vi "HW_set_IO_ports.vi"() -> ()   [LabVIEW 2016]
panel:
  out "Sync parameters cluster output":cluster{"SYNC configuration":u32}
  in  "Reset IO":bool
  in  "IO 4 zone":bool
  in  "IO 4 start/stop":bool
  in  "IO 3 zone":bool
  in  "IO 3 start/stop":bool
  in  "IO 2 sync":bool
  in  "IO 2 zone":bool=TRUE
  in  "IO 2 start/stop":bool
  in  "IO 1 sync":bool
  in  "IO 1 zone":bool=TRUE
  in  "IO 1 start/stop":bool
  in  "IO 4":u8(slide)=1 scale=0.0..1.0
  in  "IO 3":u8(slide)=1 scale=0.0..1.0
  in  "IO 2":u8(slide) scale=0.0..1.0
  in  "Exit":bool
  in  "Save Settings":bool
  in  "IO 1":u8(slide) scale=0.0..1.0
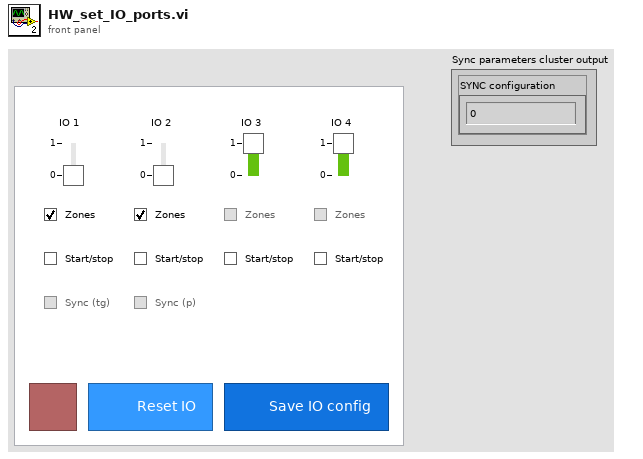
[diagram p1: front panel]
types:
  T1 = enum8{"Enabled", "Disabled", "Disabled and Grayed Out"}
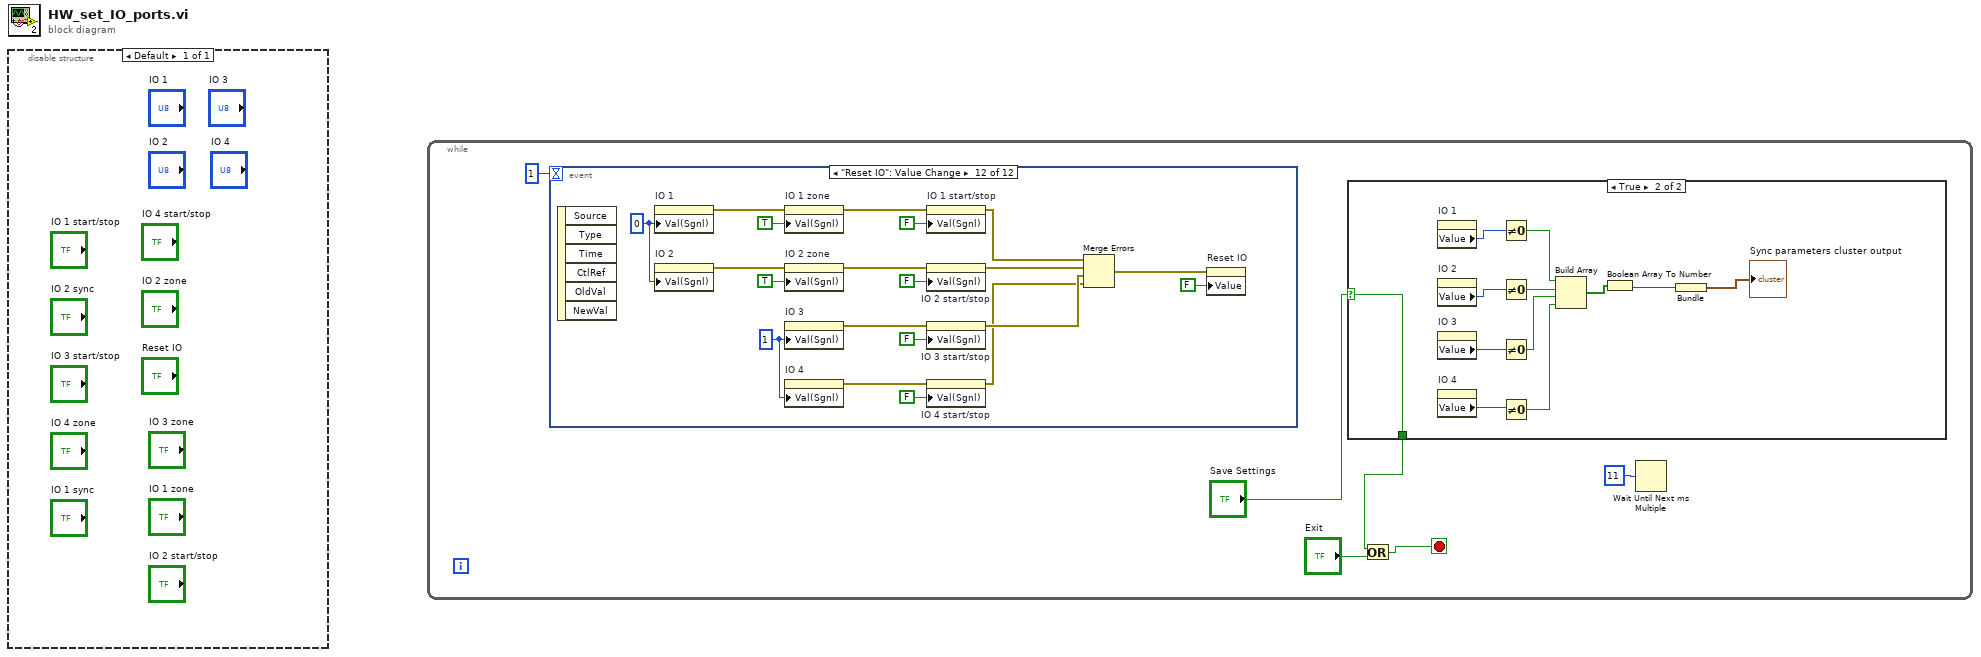
[diagram p0: block diagram]
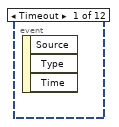
[diagram p3: hidden frame]
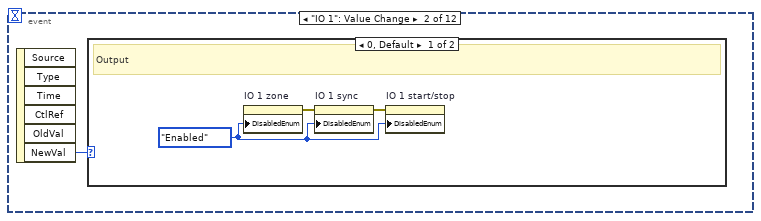
[diagram p4: hidden frame]
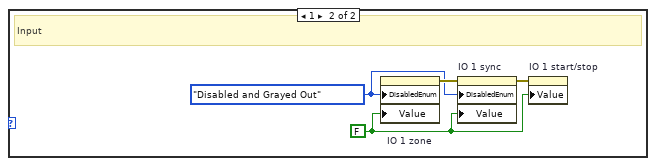
[diagram p5: hidden frame]
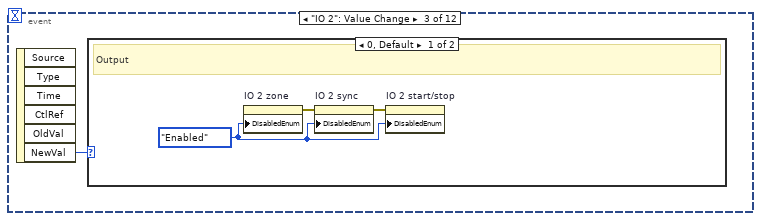
[diagram p6: hidden frame]
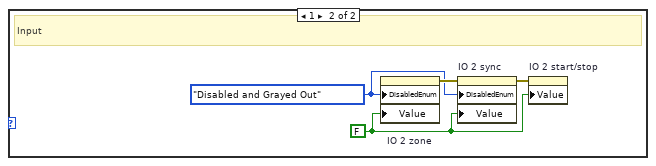
[diagram p7: hidden frame]
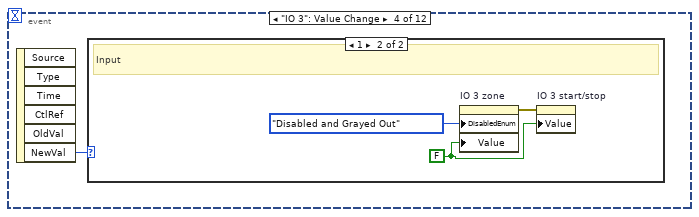
[diagram p8: hidden frame]
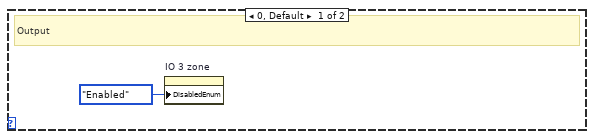
[diagram p9: hidden frame]
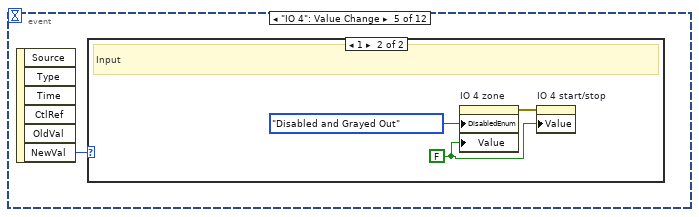
[diagram p10: hidden frame]
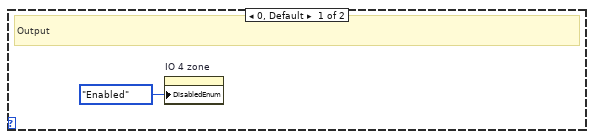
[diagram p11: hidden frame]
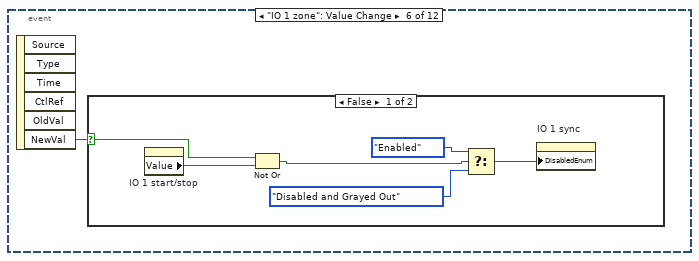
[diagram p12: hidden frame]
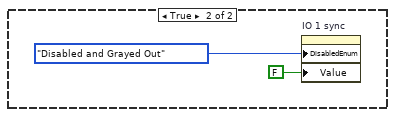
[diagram p13: hidden frame]
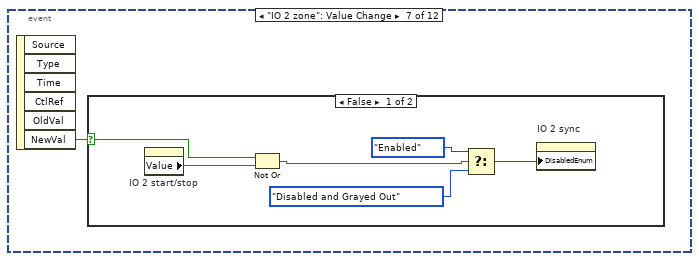
[diagram p14: hidden frame]
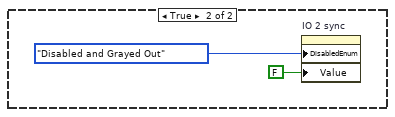
[diagram p15: hidden frame]
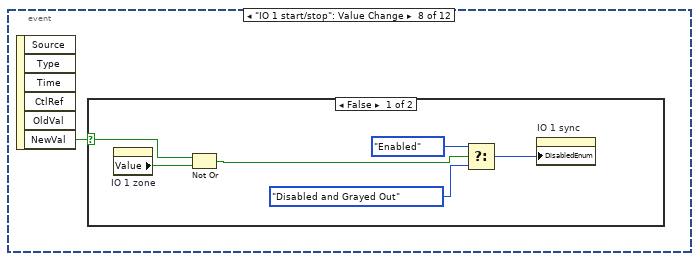
[diagram p16: hidden frame]
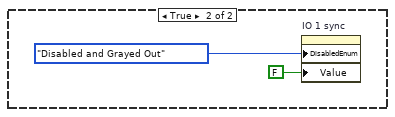
[diagram p17: hidden frame]
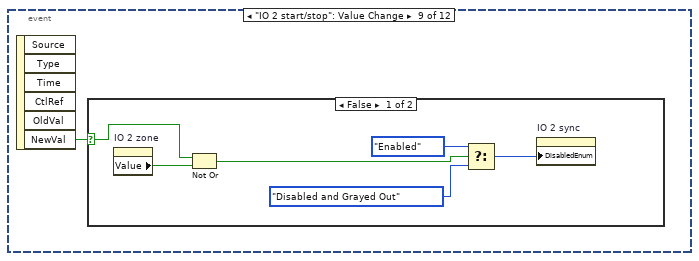
[diagram p18: hidden frame]
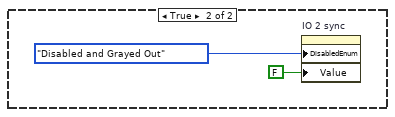
[diagram p19: hidden frame]
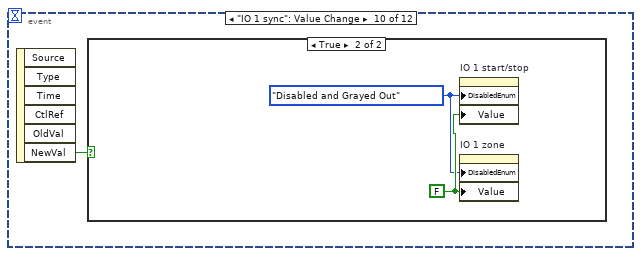
[diagram p20: hidden frame]
diagram:
  n1 = disable-structure shown="Default" {
    frame Enabled {
    }
  }
  n2 = while {
    stop <- w3 stop-if-true
    n3 = event shown="[11] \"Reset IO\": Value Change" {
      selector: _ -> [_ _ _ _ _ _ _ _ _ _ _ _]
      dyn-events: _ -> [_ _ _ _ _ _ _ _ _ _ _ _]
      timeout: 1 -> [_ _ _ _ _ _ _ _ _ _ _ _]
      event Timeout {
        n4 = event-data() -> ()  [unwired: 1 in, 3 out]
      }
      event "IO 1": Value Change {
        n5 = event-data() -> ("NewVal"=w20:u8)  [unwired: 1 in, 5 out]
        n6 = case shown="0, Default" w20 {
          frame 0, Default {
            w21 = T1."Enabled" ("Disabled")
            # "Output"
            n7 = property on="IO 1 zone" class="Bool (strict)"("DisabledEnum"=w21) -> (error out=w23:errorcluster)  [unwired: 2 in, 1 out]
            n8 = property on="IO 1 sync" class="Bool (strict)"(error in=w23, "DisabledEnum"=w21) -> (error out=w22:errorcluster)  [unwired: 1 in, 1 out]
            n9 = property on="IO 1 start/stop" class="Bool (strict)"(error in=w22, "DisabledEnum"=w21) -> ()  [unwired: 1 in, 2 out]
          }
          frame 1 {
            w24 = FALSE ("IO 1 std.")
            w26 = T1."Disabled and Grayed Out" ("Disabled")
            # "Input"
            n10 = property on="IO 1 zone" class="Bool (strict)"("DisabledEnum"=w26, "Value"=w24) -> (error out=w27:errorcluster)  [unwired: 2 in, 1 out]
            n11 = property on="IO 1 sync" class="Bool (strict)"(error in=w27, "DisabledEnum"=w26, "Value"=w24) -> (error out=w25:errorcluster)  [unwired: 1 in, 1 out]
            n12 = property on="IO 1 start/stop" class="Bool (strict)"(error in=w25, "Value"=w24) -> ()  [unwired: 1 in, 2 out]
          }
        }
      }
      event "IO 2": Value Change {
        n13 = event-data() -> ("NewVal"=w28:u8)  [unwired: 1 in, 5 out]
        n14 = case shown="0, Default" w28 {
          frame 0, Default {
            w29 = T1."Enabled" ("Disabled")
            # "Output"
            n15 = property on="IO 2 zone" class="Bool (strict)"("DisabledEnum"=w29) -> (error out=w31:errorcluster)  [unwired: 2 in, 1 out]
            n16 = property on="IO 2 sync" class="Bool (strict)"(error in=w31, "DisabledEnum"=w29) -> (error out=w30:errorcluster)  [unwired: 1 in, 1 out]
            n17 = property on="IO 2 start/stop" class="Bool (strict)"(error in=w30, "DisabledEnum"=w29) -> ()  [unwired: 1 in, 2 out]
          }
          frame 1 {
            w32 = FALSE ("IO 1 std.")
            w34 = T1."Disabled and Grayed Out" ("Disabled")
            # "Input"
            n18 = property on="IO 2 zone" class="Bool (strict)"("DisabledEnum"=w34, "Value"=w32) -> (error out=w35:errorcluster)  [unwired: 2 in, 1 out]
            n19 = property on="IO 2 sync" class="Bool (strict)"(error in=w35, "DisabledEnum"=w34, "Value"=w32) -> (error out=w33:errorcluster)  [unwired: 1 in, 1 out]
            n20 = property on="IO 2 start/stop" class="Bool (strict)"(error in=w33, "Value"=w32) -> ()  [unwired: 1 in, 2 out]
          }
        }
      }
      event "IO 3": Value Change {
        n21 = event-data() -> ("NewVal"=w36:u8)  [unwired: 1 in, 5 out]
        n22 = case shown="1" w36 {
          frame 0, Default {
            # "Output"
            n23 = property on="IO 3 zone" class="Bool (strict)"("DisabledEnum"=T1."Enabled" ("Disabled")) -> ()  [unwired: 2 in, 2 out]
          }
          frame 1 {
            w38 = FALSE ("IO 1 std.")
            # "Input"
            n24 = property on="IO 3 zone" class="Bool (strict)"("DisabledEnum"=T1."Disabled and Grayed Out" ("Disabled"), "Value"=w38) -> (error out=w39:errorcluster)  [unwired: 2 in, 1 out]
            n25 = property on="IO 3 start/stop" class="Bool (strict)"(error in=w39, "Value"=w38) -> ()  [unwired: 1 in, 2 out]
          }
        }
      }
      event "IO 4": Value Change {
        n26 = event-data() -> ("NewVal"=w41:u8)  [unwired: 1 in, 5 out]
        n27 = case shown="1" w41 {
          frame 0, Default {
            # "Output"
            n28 = property on="IO 4 zone" class="Bool (strict)"("DisabledEnum"=T1."Enabled" ("Disabled")) -> ()  [unwired: 2 in, 2 out]
          }
          frame 1 {
            w43 = FALSE ("IO 1 std.")
            # "Input"
            n29 = property on="IO 4 zone" class="Bool (strict)"("DisabledEnum"=T1."Disabled and Grayed Out" ("Disabled"), "Value"=w43) -> (error out=w44:errorcluster)  [unwired: 2 in, 1 out]
            n30 = property on="IO 4 start/stop" class="Bool (strict)"(error in=w44, "Value"=w43) -> ()  [unwired: 1 in, 2 out]
          }
        }
      }
      event "IO 1 zone": Value Change {
        n31 = event-data() -> ("NewVal"=w46:bool)  [unwired: 1 in, 5 out]
        n32 = case shown="False" w46 {
          selector: w46 -> [w51 _]
          frame False {
            n33 = property on="IO 1 start/stop" class="Bool (strict)"() -> ("Value"=w52:bool)  [unwired: 2 in, 2 out]
            n34 = Not Or(1:w52, 2:w51) -> (0:w50:bool)
            n35 = Select(t=T1."Enabled" ("Disabled"), s=w50, f=T1."Disabled and Grayed Out") -> (s? t:f=w48:T1)
            n36 = property on="IO 1 sync" class="Bool (strict)"("DisabledEnum"=w48) -> ()  [unwired: 2 in, 2 out]
          }
          frame True {
            n37 = property on="IO 1 sync" class="Bool (strict)"("DisabledEnum"=T1."Disabled and Grayed Out" ("Disabled"), "Value"=FALSE ("IO 1 sync")) -> ()  [unwired: 2 in, 2 out]
          }
        }
      }
      event "IO 2 zone": Value Change {
        n38 = event-data() -> ("NewVal"=w55:bool)  [unwired: 1 in, 5 out]
        n39 = case shown="False" w55 {
          selector: w55 -> [w60 _]
          frame False {
            n40 = property on="IO 2 start/stop" class="Bool (strict)"() -> ("Value"=w61:bool)  [unwired: 2 in, 2 out]
            n41 = Not Or(1:w61, 2:w60) -> (0:w59:bool)
            n42 = Select(t=T1."Enabled" ("Disabled"), s=w59, f=T1."Disabled and Grayed Out") -> (s? t:f=w57:T1)
            n43 = property on="IO 2 sync" class="Bool (strict)"("DisabledEnum"=w57) -> ()  [unwired: 2 in, 2 out]
          }
          frame True {
            n44 = property on="IO 2 sync" class="Bool (strict)"("DisabledEnum"=T1."Disabled and Grayed Out" ("Disabled"), "Value"=FALSE ("IO 1 sync")) -> ()  [unwired: 2 in, 2 out]
          }
        }
      }
      event "IO 1 start/stop": Value Change {
        n45 = event-data() -> ("NewVal"=w64:bool)  [unwired: 1 in, 5 out]
        n46 = case shown="False" w64 {
          selector: w64 -> [w70 _]
          frame False {
            n47 = property on="IO 1 zone" class="Bool (strict)"() -> ("Value"=w69:bool)  [unwired: 2 in, 2 out]
            n48 = Not Or(1:w69, 2:w70) -> (0:w68:bool)
            n49 = Select(t=T1."Enabled" ("Disabled"), s=w68, f=T1."Disabled and Grayed Out") -> (s? t:f=w65:T1)
            n50 = property on="IO 1 sync" class="Bool (strict)"("DisabledEnum"=w65) -> ()  [unwired: 2 in, 2 out]
          }
          frame True {
            n51 = property on="IO 1 sync" class="Bool (strict)"("DisabledEnum"=T1."Disabled and Grayed Out" ("Disabled"), "Value"=FALSE ("IO 1 sync")) -> ()  [unwired: 2 in, 2 out]
          }
        }
      }
      event "IO 2 start/stop": Value Change {
        n52 = event-data() -> ("NewVal"=w73:bool)  [unwired: 1 in, 5 out]
        n53 = case shown="False" w73 {
          selector: w73 -> [w79 _]
          frame False {
            n54 = property on="IO 2 zone" class="Bool (strict)"() -> ("Value"=w78:bool)  [unwired: 2 in, 2 out]
            n55 = Not Or(1:w78, 2:w79) -> (0:w77:bool)
            n56 = Select(t=T1."Enabled" ("Disabled"), s=w77, f=T1."Disabled and Grayed Out") -> (s? t:f=w74:T1)
            n57 = property on="IO 2 sync" class="Bool (strict)"("DisabledEnum"=w74) -> ()  [unwired: 2 in, 2 out]
          }
          frame True {
            n58 = property on="IO 2 sync" class="Bool (strict)"("DisabledEnum"=T1."Disabled and Grayed Out" ("Disabled"), "Value"=FALSE ("IO 1 sync")) -> ()  [unwired: 2 in, 2 out]
          }
        }
      }
      event "IO 1 sync": Value Change {
        n59 = event-data() -> ("NewVal"=w82:bool)  [unwired: 1 in, 5 out]
        n60 = case shown="True" w82 {
          frame False {
            w84 = T1."Enabled" ("Disabled")
            n61 = property on="IO 1 zone" class="Bool (strict)"("DisabledEnum"=w84) -> (error out=w83:errorcluster)  [unwired: 2 in, 1 out]
            n62 = property on="IO 1 start/stop" class="Bool (strict)"(error in=w83, "DisabledEnum"=w84) -> ()  [unwired: 1 in, 2 out]
          }
          frame True {
            w85 = T1."Disabled and Grayed Out" ("Disabled")
            w86 = FALSE ("IO 1 zone")
            n63 = property on="IO 1 start/stop" class="Bool (strict)"("DisabledEnum"=w85, "Value"=w86) -> ()  [unwired: 2 in, 2 out]
            n64 = property on="IO 1 zone" class="Bool (strict)"("DisabledEnum"=w85, "Value"=w86) -> ()  [unwired: 2 in, 2 out]
          }
        }
      }
      event "IO 2 sync": Value Change {
        n65 = event-data() -> ("NewVal"=w87:bool)  [unwired: 1 in, 5 out]
        n66 = case shown="False" w87 {
          frame False {
            w89 = T1."Enabled" ("Disabled")
            n67 = property on="IO 2 zone" class="Bool (strict)"("DisabledEnum"=w89) -> (error out=w88:errorcluster)  [unwired: 2 in, 1 out]
            n68 = property on="IO 2 start/stop" class="Bool (strict)"(error in=w88, "DisabledEnum"=w89) -> ()  [unwired: 1 in, 2 out]
          }
          frame True {
            w90 = T1."Disabled and Grayed Out" ("Disabled")
            w91 = FALSE ("IO 1 zone")
            n69 = property on="IO 2 start/stop" class="Bool (strict)"("DisabledEnum"=w90, "Value"=w91) -> ()  [unwired: 2 in, 2 out]
            n70 = property on="IO 2 zone" class="Bool (strict)"("DisabledEnum"=w90, "Value"=w91) -> ()  [unwired: 2 in, 2 out]
          }
        }
      }
      event "Reset IO": Value Change {
        w110 = u8 1 ("Value (Signaling)")
        w111 = u8 0 ("Value (Signaling)")
        n71 = event-data() -> ()  [unwired: 1 in, 6 out]
        n72 = property on="IO 1" class="Slide (strict)"("Val(Sgnl)"=w111) -> (error out=w109:errorcluster)  [unwired: 2 in, 1 out]
        n73 = property on="IO 2" class="Slide (strict)"("Val(Sgnl)"=w111) -> (error out=w102:errorcluster)  [unwired: 2 in, 1 out]
        n74 = property on="IO 1 zone" class="Bool (strict)"(error in=w109, "Val(Sgnl)"=TRUE ("Value (Signaling)")) -> (error out=w108:errorcluster)  [unwired: 1 in, 1 out]
        n75 = property on="IO 2 zone" class="Bool (strict)"(error in=w102, "Val(Sgnl)"=TRUE ("Value (Signaling)")) -> (error out=w103:errorcluster)  [unwired: 1 in, 1 out]
        n76 = property on="IO 3" class="Slide (strict)"("Val(Sgnl)"=w110) -> (error out=w100:errorcluster)  [unwired: 2 in, 1 out]
        n77 = property on="IO 4" class="Slide (strict)"("Val(Sgnl)"=w110) -> (error out=w98:errorcluster)  [unwired: 2 in, 1 out]
        n78 = property on="IO 1 start/stop" class="Bool (strict)"(error in=w108, "Val(Sgnl)"=FALSE ("Value (Signaling)")) -> (error out=w97:errorcluster)  [unwired: 1 in, 1 out]
        n79 = property on="IO 2 start/stop" class="Bool (strict)"(error in=w103, "Val(Sgnl)"=FALSE ("Value (Signaling)")) -> (error out=w96:errorcluster)  [unwired: 1 in, 1 out]
        n80 = property on="IO 3 start/stop" class="Bool (strict)"(error in=w100, "Val(Sgnl)"=FALSE ("Value (Signaling)")) -> (error out=w95:errorcluster)  [unwired: 1 in, 1 out]
        n81 = property on="IO 4 start/stop" class="Bool (strict)"(error in=w98, "Val(Sgnl)"=FALSE ("Value (Signaling)")) -> (error out=w94:errorcluster)  [unwired: 1 in, 1 out]
        n82 = Merge Errors(w97, w96, w95, w94) -> (w93:errorcluster)
        n83 = property on="Reset IO" class="Bool (strict)"(error in=w93, "Value"=FALSE ("Reset IO")) -> ()  [unwired: 1 in, 2 out]
      }
    }
    n84 = case shown="True" "Save Settings" {
      selector: "Save Settings" -> [w7 w8]
      tunnel: [w7 w8] -> w1
      frame False {
      }
      frame True {
        n85 = property on="IO 1" class="Slide (strict)"() -> ("Value"=w19:u8)  [unwired: 2 in, 2 out]
        n86 = property on="IO 2" class="Slide (strict)"() -> ("Value"=w18:u8)  [unwired: 2 in, 2 out]
        n87 = property on="IO 3" class="Slide (strict)"() -> ("Value"=w17:u8)  [unwired: 2 in, 2 out]
        n88 = property on="IO 4" class="Slide (strict)"() -> ("Value"=w16:u8)  [unwired: 2 in, 2 out]
        n89 = Not Equal To 0?(x=w19) -> (x != 0?=w15:bool)
        n90 = Not Equal To 0?(x=w18) -> (x != 0?=w14:bool)
        n91 = Not Equal To 0?(x=w17) -> (x != 0?=w13:bool)
        n92 = Not Equal To 0?(x=w16) -> (x != 0?=w12:bool)
        n93 = Build Array(w15, w14, w13, w12) -> (w11:bool[])
        n94 = Boolean Array To Number(Boolean array=w11) -> (number=w10:u32)
        n95 = Bundle(w10) -> (→"Sync parameters cluster output":cluster{u32})  [unwired: 1 in]
      }
    }
    n96 = Or(x=w1, y="Exit") -> (x .or. y?=w3:bool)
    n97 = Wait Until Next ms Multiple(millisecond multiple=u32 11) -> ()  [unwired: 1 out]
  }
